vi "DriveWait.vi"(2 "Parameter String":string, 3 "Reinit":bool) -> (0 "Error Out":errorcluster, 1 "Increment":bool)   [LabVIEW 2019]
doc: "This VI pauses the drive sequencer until the specified condition is met. Four different modes are available: time_delay, sequencer_step, time_since_shooter, and balls_shot.\n\nParameters:\ntime_delay --> wait for param1{time delay (ms) or if -1 from the dashboard (s)}, param2{1}\nsequencer_step --> wait for param1{subsytem sequence step (#)}, param2{1}\ntime_since_shooter --> wait for param1{time (ms)} since shooter started shooting, param2{1}\nmode=balls_shot --> wait for param2{current balls shot} or until param1{timeout(ms), set to -1 to ignore}"
uses:
  SafeParser_Integer.vi
  dscommands.vi
  dsdata.vi
  autoninfo.vi
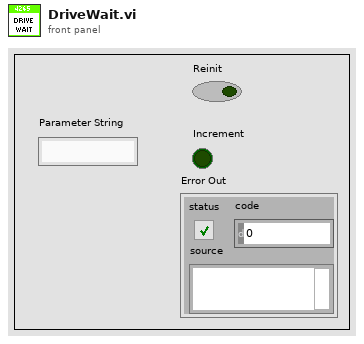
[diagram p1: front panel]
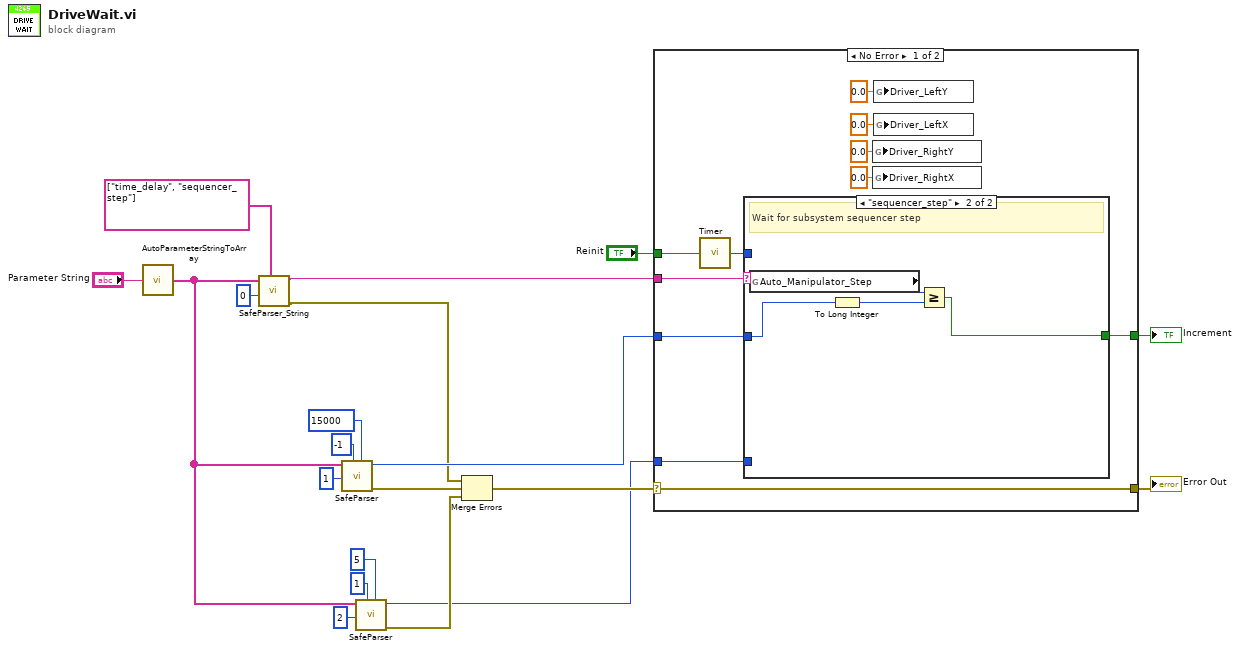
[diagram p0: block diagram]
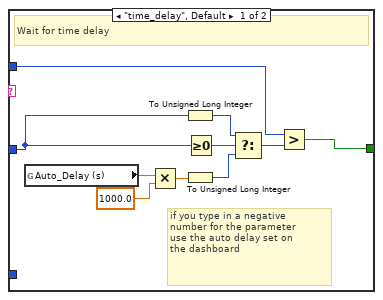
[diagram p2: hidden frame]
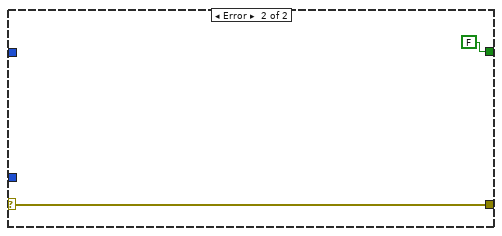
[diagram p3: hidden frame]
diagram:
  n1 = call "AutoParameterStringToArray.vi"("Parameter String"="Parameter String") -> ("Parsed Parameters"=w4:string[])
  n2 = call "SafeParser_String.vi"("Allowed Values"=string[] ["time_delay", "sequencer_step"], "Array Index"=0, "String Array"=w4) -> ("Error Out"=w8:errorcluster, "Typecast Value"=w9:string)  [unwired: 7 in]
  n3 = call-poly "SafeParser.vi"("Maximum"=15000, "Minimum"=-1, "Array Index"=1 ("Parameter Index"), "String Array"=w4) -> ("Error Out"=w16:errorcluster, "Typecast  Value"=w14:i32)  [unwired: 6 in]
  n4 = call-poly "SafeParser.vi"("Maximum"=5, "Minimum"=1, "Array Index"=2 ("Parameter Index"), "String Array"=w4) -> ("Error Out"=w3:errorcluster, "Typecast  Value"=w2:i32)  [unwired: 6 in]
  n5 = Merge Errors(w8, w16, w3) -> (w15:errorcluster)
  n6 = case shown="No Error" w15 {
    selector: w15 -> [w23 w47]
    tunnel: w9 -> [w27 _]
    tunnel: [w26 FALSE] -> w20
    tunnel: "Reinit" -> [w25 _]
    tunnel: [w23 w47] -> w18
    tunnel: w14 -> [w22 _]
    tunnel: w2 -> [w21 _]
    frame No Error {
      n7 = call "Timer.vi"("Reset Timer"=w25) -> ("Time (ms)"=w24:u32)
      n8 = case shown="\"sequencer_step\"" w27 {
        tunnel: w24 -> [w34 _]
        tunnel: [w33 w43] -> w26
        tunnel: w22 -> [w32 w42]
        tunnel: w21 -> [_ _]
        frame "time_delay", Default {
          # "if you type in a negative\nnumber for the parameter\nuse the auto delay set on \nthe dashboard"
          # "Wait for time delay"
          n9 = global read "dsdata.vi" "Auto_Delay (s)"() -> (w39:dbl)
          n10 = Multiply(x=w39, y=1000.0) -> (x*y=w40:dbl)
          n11 = To Unsigned Long Integer(number=w32) -> (unsigned 32bit integer=w38:u32)
          n12 = To Unsigned Long Integer(number=w40) -> (unsigned 32bit integer=w41:u32)
          n13 = Greater Or Equal To 0?(x=w32) -> (x >= 0?=w37:bool)
          n14 = Select(t=w38, s=w37, f=w41) -> (s? t:f=w35:u32)
          n15 = Greater?(x=w34, y=w35) -> (0:w33:bool)
        }
        frame "sequencer_step" {
          # "Wait for subsystem sequencer step"
          n16 = global read "autoninfo.vi" "Auto_Manipulator_Step"() -> (w45:i32)
          n17 = To Long Integer(number=w42) -> (32bit integer=w44:i32)
          n18 = Greater Or Equal?(x=w45, y=w44) -> (x >= y?=w43:bool)
        }
      }
      n19 = global write "dscommands.vi" "Driver_RightY"(0.0 ("Driver_RightX")) -> ()
      n20 = global write "dscommands.vi" "Driver_RightX"(0.0 ("Driver_RightX")) -> ()
      n21 = global write "dscommands.vi" "Driver_LeftY"(0.0 ("Driver_LeftY")) -> ()
      n22 = global write "dscommands.vi" "Driver_LeftX"(0.0 ("Driver_RightX")) -> ()
    }
    frame Error {
    }
  }
  "Increment" <- w20
  "Error Out" <- w18
